vi "Paths Reorder.vi"(9 "Display State In":T2 caption="显示状态输入", 10 "Enum":enum16{"Move Up", "Move Down"}(ring) caption="枚举", 11 "Include Paths Ref":refnum<vi> caption="包括路径引用") -> (1 "Display State Out":T2 caption="显示状态输出", 2 "Path Strings Out":T1 caption="路径字符串输出", 3 "Dup Include Paths Ref":refnum<vi> caption="包括路径引用副本")   [LabVIEW 2011, in "NISAST Include Paths.xctl"]
uses:
  NISAST Include Paths.xctl
  State.ctl
  Data.ctl
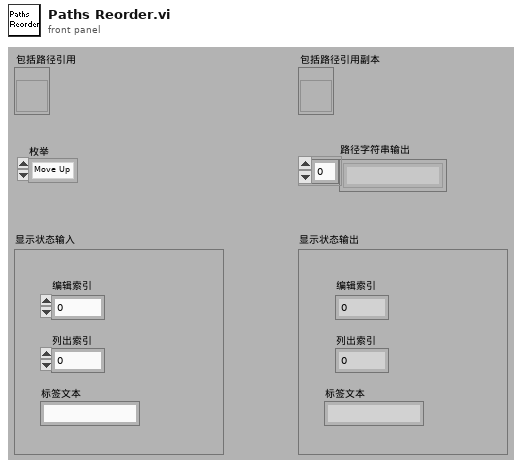
[diagram p1: front panel]
types:
  T1 = typedef "NISAST Include Paths.xctl/Data.ctl" = string[]
  T2 = typedef "NISAST Include Paths.xctl/State.ctl" = cluster{"Edit Index":i32, "List Index":i32, "Label Text":string}
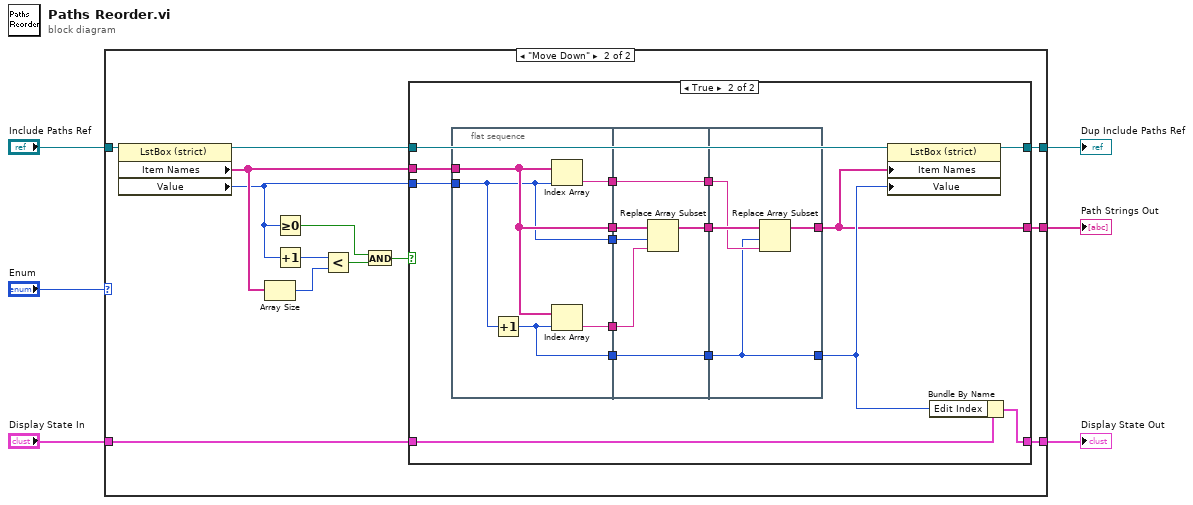
[diagram p0: block diagram]
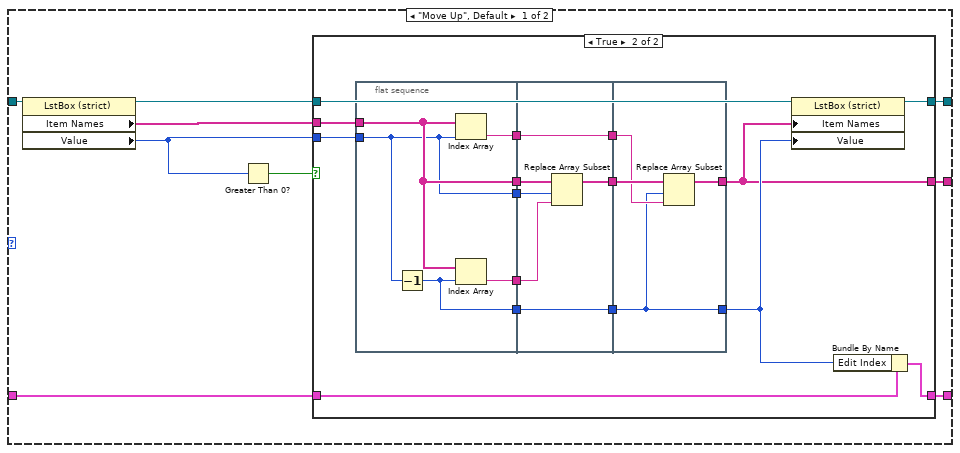
[diagram p2: hidden frame]
diagram:
  n1 = case shown="\"Move Down\"" "Enum" {
    tunnel: "Include Paths Ref" -> [w13 w62]
    tunnel: "Display State In" -> [w11 w61]
    tunnel: [w10 w60] -> w4
    tunnel: [w12 w58] -> w3
    tunnel: [w7 w54] -> w1
    frame "Move Up", Default {
      n2 = property class="LstBox (strict)"(reference=w13) -> (reference out=w15:refnum<vi>, "Item Names"=w14:string[], "Value"=w9:i32)  [unwired: 1 in, 1 out]
      n3 = Greater Than 0?(x=w9) -> (x > 0?=w8:bool)
      n4 = case shown="True" w8 {
        tunnel: w15 -> [w18 w26]
        tunnel: w9 -> [_ w25]
        tunnel: w14 -> [w16 w24]
        tunnel: [w18 w23] -> w12
        tunnel: w11 -> [w17 w22]
        tunnel: [w17 w21] -> w10
        tunnel: [w16 w19] -> w7
        frame False {
        }
        frame True {
          n5 = flat-sequence {
            tunnel: w24 -> [w39]
            tunnel: w25 -> [w37]
            tunnel: [w39] -> w34
            tunnel: [w38] -> w33
            tunnel: [w37] -> w32
            tunnel: [w36] -> w31
            tunnel: [w35] -> w30
            tunnel: w34 -> [w45]
            tunnel: w33 -> [w44]
            tunnel: w32 -> [w43]
            tunnel: [w42] -> w29
            tunnel: w31 -> [w41]
            tunnel: [w41] -> w28
            tunnel: w30 -> [w40]
            tunnel: [w40] -> w27
            tunnel: w29 -> [w49]
            tunnel: w28 -> [w47]
            tunnel: w27 -> [w48]
            tunnel: [w47] -> w20
            tunnel: [w46] -> w19
            frame #0 {
              n6 = Decrement(x=w37) -> (x-1=w36:i32)
              n7 = Index Array(array=w39, index=w37) -> (element=w35:string)
              n8 = Index Array(array=w39, index=w36) -> (element=w38:string)
            }
            frame #1 {
              n9 = Replace Array Subset(array=w45, new element=w44, index=w43) -> (w42:string[])
            }
            frame #2 {
              n10 = Replace Array Subset(array=w49, new element=w48, index=w47) -> (w46:string[])
            }
          }
          n11 = property class="LstBox (strict)"(reference=w26, "Item Names"=w19, "Value"=w20) -> (reference out=w23:refnum<vi>)  [unwired: 1 in, 1 out]
          n12 = Bundle By Name(cluster=w22, "Edit Index"=w20) -> (w21:T2)
        }
      }
    }
    frame "Move Down" {
      n13 = property class="LstBox (strict)"(reference=w62) -> (reference out=w59:refnum<vi>, "Item Names"=w57:string[], "Value"=w53:i32)  [unwired: 1 in, 1 out]
      n14 = Array Size(array=w57) -> (size(s)=w56:i32)
      n15 = Greater Or Equal To 0?(x=w53) -> (x >= 0?=w51:bool)
      n16 = Increment(x=w53) -> (x+1=w55:i32)
      n17 = Less?(x=w55, y=w56) -> (x < y?=w52:bool)
      n18 = And(x=w51, y=w52) -> (x .and. y?=w50:bool)
      n19 = case shown="True" w50 {
        tunnel: w57 -> [w63 w73]
        tunnel: w53 -> [_ w72]
        tunnel: w61 -> [w64 w71]
        tunnel: [w64 w70] -> w60
        tunnel: w59 -> [w65 w69]
        tunnel: [w65 w68] -> w58
        tunnel: [w63 w66] -> w54
        frame False {
        }
        frame True {
          n20 = flat-sequence {
            tunnel: w73 -> [w86]
            tunnel: w72 -> [w84]
            tunnel: [w86] -> w81
            tunnel: [w85] -> w80
            tunnel: [w84] -> w79
            tunnel: [w83] -> w78
            tunnel: [w82] -> w77
            tunnel: w81 -> [w92]
            tunnel: w80 -> [w91]
            tunnel: w79 -> [w90]
            tunnel: [w89] -> w76
            tunnel: w78 -> [w88]
            tunnel: [w88] -> w75
            tunnel: w77 -> [w87]
            tunnel: [w87] -> w74
            tunnel: w76 -> [w96]
            tunnel: w75 -> [w94]
            tunnel: w74 -> [w95]
            tunnel: [w94] -> w67
            tunnel: [w93] -> w66
            frame #0 {
              n21 = Increment(x=w84) -> (x+1=w83:i32)
              n22 = Index Array(array=w86, index=w84) -> (element=w82:string)
              n23 = Index Array(array=w86, index=w83) -> (element=w85:string)
            }
            frame #1 {
              n24 = Replace Array Subset(array=w92, new element=w91, index=w90) -> (w89:string[])
            }
            frame #2 {
              n25 = Replace Array Subset(array=w96, new element=w95, index=w94) -> (w93:string[])
            }
          }
          n26 = property class="LstBox (strict)"(reference=w69, "Item Names"=w66, "Value"=w67) -> (reference out=w68:refnum<vi>)  [unwired: 1 in, 1 out]
          n27 = Bundle By Name(cluster=w71, "Edit Index"=w67) -> (w70:T2)
        }
      }
    }
  }
  "Display State Out" <- w4
  "Dup Include Paths Ref" <- w3
  "Path Strings Out" <- w1
